vi "Do.vi"(8 "error in (no error)":errorcluster, 10 "Actor in":refnum<class "Actor.lvclass">, 11 "MoveBySteps Msg":refnum<class "MoveBySteps Msg.lvclass">) -> (0 "error out":errorcluster, 2 "Actor out":refnum<class "Actor.lvclass">)   [LabVIEW 2023, in "MoveBySteps Msg.lvclass"]
doc: "This VI delivers the message to the actor by calling the appropriate method(s) on the actor."
uses:
  MoveBySteps Msg.lvclass
  MoveBySteps Msg.lvclass/MoveBySteps Msg.ctl
  9ef47adc-f318-494c-9b8b-6df3216d6863.vi
  TranslationStages/TranslationStages.lvclass
  <vilib>/ActorFramework/Actor/Actor.lvclass
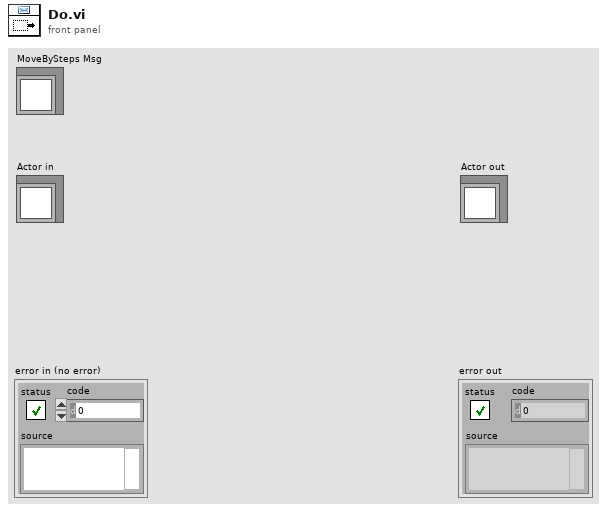
[diagram p1: front panel]
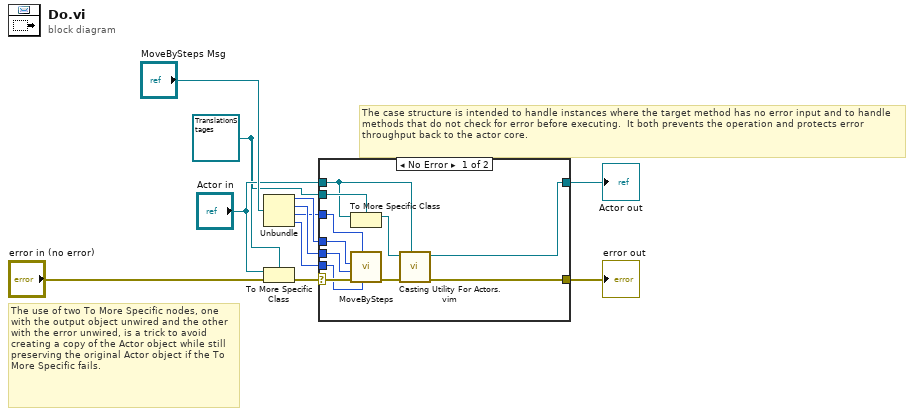
[diagram p0: block diagram]
diagram:
  w5 = refnum<class "TranslationStages.lvclass"> refnum ("Actor in")
  # "The use of two To More Specific nodes, one with the output object unwired and the other with the error unwired, is a trick to avoid creating a copy of the Actor object while still preserving the original Actor object if the To More Specific fails."
  # "The case structure is intended to handle instances where the target method has no error input and to handle methods that do not check for error before executing.  It both prevents the operation and protects error throughput back to the actor core."
  n1 = Unbundle("MoveBySteps Msg") -> (w4:u32, w3:u32, w2:enum16{"Positive", "Negative"}, w1:enum16{"Forward", "Backwards"})
  n2 = To More Specific Class(target class=w5, reference="Actor in", error in="error in (no error)") -> (error out=w9:errorcluster)  [unwired: 1 out]
  n3 = case shown="No Error" w9 {
    selector: w9 -> [w22 w24]
    tunnel: [w17 w24] -> w8
    tunnel: [w18 w23] -> w7
    tunnel: "Actor in" -> [w19 w23]
    tunnel: w5 -> [w20 _]
    tunnel: w4 -> [w15 _]
    tunnel: w3 -> [w14 _]
    tunnel: w2 -> [w13 _]
    tunnel: w1 -> [w12 _]
    frame No Error {
      n4 = To More Specific Class(target class=w20, reference=w19) -> (specific class reference=w21:refnum<class "TranslationStages.lvclass">)  [unwired: 1 in, 1 out]
      n5 = call "MoveBySteps.vi"("Direction"=w12, "Polarity"=w13, "error in (no error)"=w22, "Speed"=w14, "Steps"=w15) -> ("error out"=w16:errorcluster)  [unwired: 6 in]
      n6 = call "Casting Utility For Actors.vim"("type"=w19, "error in (no error)"=w16, "Actor in"=w21) -> ("error out"=w17:errorcluster, "Actor out"=w18:refnum<class "Actor.lvclass">)  [unwired: 7 in]
    }
    frame Error {
      # "If type check fails, pass the original object out again."
    }
  }
  "error out" <- w8
  "Actor out" <- w7
